vi "SVD ReadVTSize.vi"(8 "error in (no error)":errorcluster, 11 "SVD in":refnum<class "SVD.lvclass">) -> (0 "error out":errorcluster, 1 "Rows":i32, 2 "Cols":i32, 3 "SVD out":refnum<class "SVD.lvclass">, 4 "Datatype":T1)   [LabVIEW 2020, in "OpenLvVision_OpenCv.lvlib" / "SVD.lvclass"]
uses:
  SVD.lvclass
  _LvHelpers/EdvrObject/EdvrObject.lvclass
  C:/Users/lukas/Downloads/OpenLvVision_OpenCv/SourceCode/LabView/OpenLvVision_OpenCv/_LvHelpers/EdvrObject/EdvrObject.lvclass
  C:/Users/lukas/Downloads/OpenLvVision_OpenCv/SourceCode/LabView/OpenLvVision_OpenCv/CoreFunctionality/SVD/SVD/SVD.lvclass
  Dlls/OlvOpenCvWrapper.dll
  TypeDef/LvDatatype.ctl
  OpenLvVision_OpenCv.lvlib
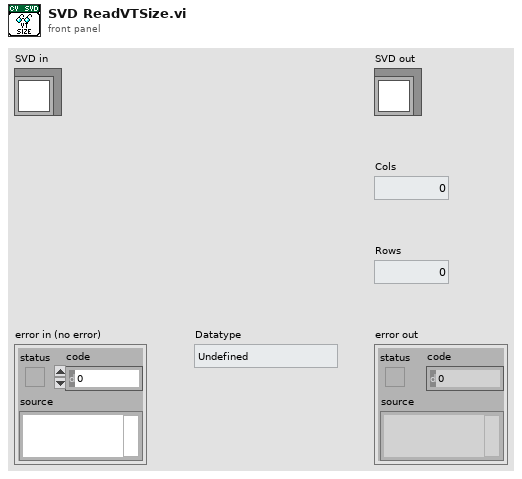
[diagram p1: front panel]
types:
  T1 = typedef "OpenLvVision_OpenCv.lvlib/LvDatatype.ctl" = enum32{"Undefined", "U8", "I8", "U16", "I16", "U32_Color", "I32", "U64_Color", "I64", "SGL", "DBL", "Complex SGL", "Complex DBL", "Array 1D U8", "Array 1D I8", "Array 1D U16", "Array 1D I16", "Array 1D U32_Color", "Array 1D I32", "Array 1D U64_Color", "Array 1D I64", "Array 1D SGL", "Array 1D DBL", "Array 1D Complex SGL", "Array 1D Complex DBL", "Array 2D U8", "Array 2D I8", "Array 2D U16", "Array 2D I16", "Array 2D U32", "Array 2D U32_Color", "Array 2D I32", "Array 2D U64", "Array 2D U64_Color", "Array 2D I64", "Array 2D SGL", "Array 2D DBL", "Array 2D Complex SGL", "Array 2D Complex DBL", "Image Mono U8", "Image Mono U16", "Image Mono I16", "Image Mono SGL", "Image Color U32", "Image Color U64", "ImageComplex Sgl", "Array1d_2dPointI32", "Array1d_2dPointSGL", "Array1d_2dPointDBL", "Array1d_3dPointI32", "Array1d_3dPointSGL", "Array1d_3dPointDBL", "Array1d_4dPointI32", "Array1d_4dPointSGL", "Array1d_4dPointDBL"}
  T2 = typedef "OpenLvVision_OpenCv.lvlib/EdvrObject.lvclass/Edvr.ctl" = refnum<data-value>
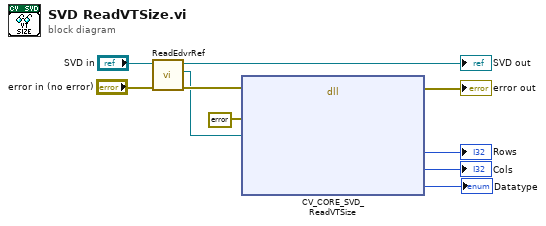
[diagram p0: block diagram]
diagram:
  n1 = call "ReadEdvrRef.vi"("error in (no error)"="error in (no error)", "EdvrObject in"="SVD in") -> ("error out"=w10:errorcluster, "Edvr"=w5:T2, "EdvrObject out"=→"SVD out":refnum<class "SVD.lvclass">)  [unwired: 7 in]
  n2 = dll-call lib="C:/Users/lukas/Downloads/OpenLvVision_OpenCv/SourceCode/LabView/OpenLvVision_OpenCv/Dlls/OlvOpenCvWrapper.dll" fn="CV_CORE_SVD_ReadVTSize"(error in=w10, "Error"=errorcluster {"status"=FALSE, "code"=0, "source"=""} ("error out"), "edvrRef"=w5) -> (error out=→"error out":errorcluster, "rows"=→"Rows":i32, "cols"=→"Cols":i32, "type"=→"Datatype":u32)  [unwired: 8 in, 1 out]
